vi "array-interpolation.vi"(1 "N Times Interpolation":i32, 2 "Interpolation Method":i32, 3 "2D Data":dbl[][](array[numeric])) -> (0 "Interpolated Data":dbl[][](array[numeric]))   [LabVIEW 2021]
uses:
  <vilib>/Analysis/1siggen.llb/Ramp Pattern by Samples.vi
  <vilib>/gmath/interp.llb/Interpolate 2D (1d xi,yi).vi
  <vilib>/Analysis/NI_AALBase.lvlib
  <vilib>/gmath/NI_Gmath.lvlib
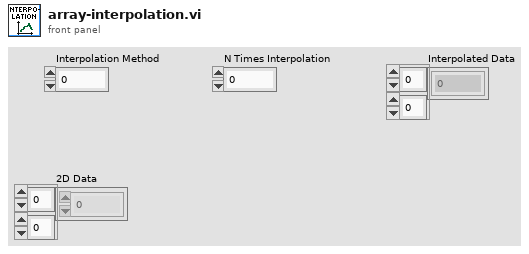
[diagram p1: front panel]
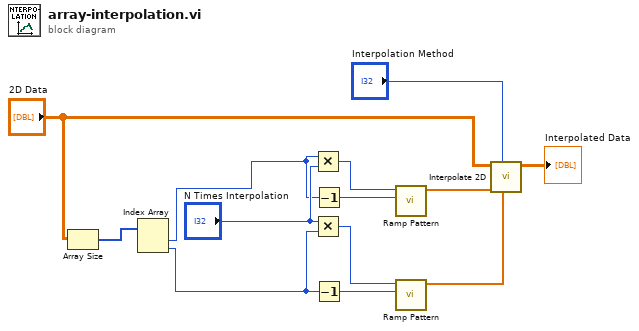
[diagram p0: block diagram]
diagram:
  n1 = Array Size(array="2D Data") -> (size(s)=w3:i32[])
  n2 = Index Array(array=w3) -> (element #1=w2:i32, element #2=w1:i32)  [unwired: 2 in]
  n3 = Multiply(x=w2, y="N Times Interpolation") -> (x*y=w7:i32)
  n4 = Multiply(x="N Times Interpolation", y=w1) -> (x*y=w8:i32)
  n5 = Decrement(x=w2) -> (x-1=w5:i32)
  n6 = Decrement(x=w1) -> (x-1=w6:i32)
  n7 = call-poly <vilib>:"Ramp Pattern.vi"("end"=w5, "samples"=w7) -> ("Ramp Pattern"=w10:dbl[])  [unwired: 8 in, 1 out]
  n8 = call-poly <vilib>:"Ramp Pattern.vi"("end"=w6, "samples"=w8) -> ("Ramp Pattern"=w11:dbl[])  [unwired: 8 in, 1 out]
  n9 = call-poly <vilib>:"Interpolate 2D.vi"("yi"=w11, "method"="Interpolation Method", "xi"=w10, "Z"="2D Data") -> ("zi"=→"Interpolated Data":dbl[][])  [unwired: 4 in, 3 out]
